vi "Calling VI.vi"() -> ()   [LabVIEW 2014]
uses:
  Integer Mean.vi
  Double Mean.vi
panel:
  in  "Stop Button":bool
  out "Integer  Mean":i64
  out "Double Mean":dbl
  in  "Byte Array":u8[](array[numeric])
  in  "Double Array":dbl[](array[numeric])
  # "Polymorphic VI"
  # "Double Array"
  # "Byte Array"
  # "Double Mean"
  # "Integer Mean"
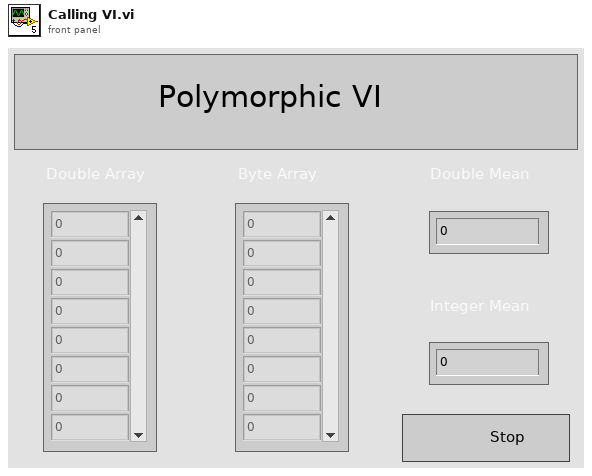
[diagram p1: front panel]
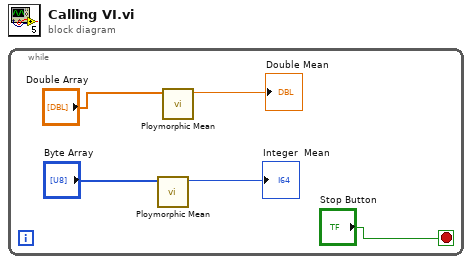
[diagram p0: block diagram]
diagram:
  n1 = while {
    stop <- "Stop Button" stop-if-true
    n2 = call-poly "Ploymorphic Mean.vi"("Integer Array"="Byte Array") -> ("Numeric"=→"Integer  Mean":i64)  [unwired: 10 in]
    n3 = call-poly "Ploymorphic Mean.vi"("Double Array"="Double Array") -> ("Numeric"=→"Double Mean":dbl)  [unwired: 10 in]
  }
